vi "Collapse Right Pane.vi"(8 "error in (no error)":errorcluster, 10 "Splitter 6":refnum<vi>, 11 "VI in":refnum<vi>) -> (0 "error out":errorcluster)   [LabVIEW 2013, in "main.lvlib"]
uses:
  main.lvlib
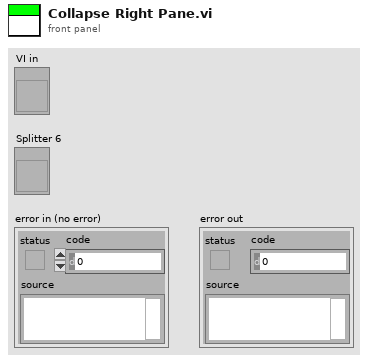
[diagram p1: front panel]
types:
  T1 = typedef "LVRectTypeDef.ctl" = cluster{"Left":i16, "Top":i16, "Right":i16, "Bottom":i16}
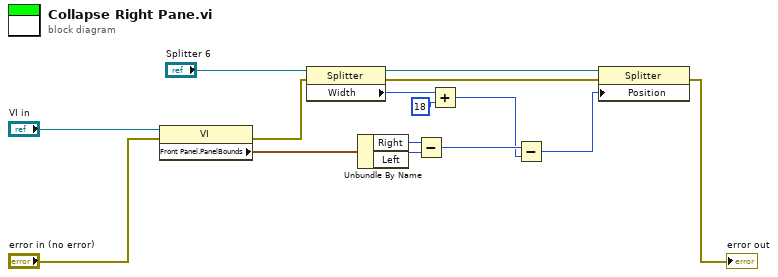
[diagram p0: block diagram]
diagram:
  n1 = property class="VI"(reference="VI in", error in="error in (no error)") -> (error out=w4:errorcluster, "Front Panel.PanelBounds"=w10:T1)  [unwired: 1 out]
  n2 = property class="Splitter"(reference="Splitter 6", error in=w4) -> (reference out=w3:refnum<vi>, error out=w1:errorcluster, "Width"=w14:u32)
  n3 = Unbundle By Name(w10) -> ("Right"=w12:i16, "Left"=w11:i16)
  n4 = Subtract(x=w12, y=w11) -> (x-y=w7:i16)
  n5 = Add(x=w14, y=u32 18) -> (x+y=w6:u32)
  n6 = Subtract(x=w7, y=w6) -> (x-y=w5:u32)
  n7 = property class="Splitter"(reference=w3, error in=w1, "Position"=w5) -> (error out=→"error out":errorcluster)  [unwired: 1 out]
